vi "Display Module Refresh Rate.vi"(7 "Refresh Rate In":u32) -> (8 "Refresh Rate Out":u32)   [LabVIEW 2020]
uses:
  <vilib>/Utility/miscctls.llb/LVPointTypeDef.ctl
panel:
  in  "Refresh Rate (ms)":u32
  in  "Cancel":bool
  in  "Okay":bool
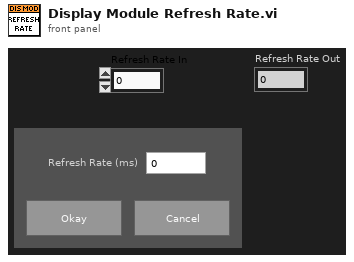
[diagram p1: front panel]
types:
  T1 = enum16{"Always On", "Always Off", "Off While Running"}
  T2 = typedef "LVPointTypeDef.ctl" = cluster{"Horizontal":i16, "Vertical":i16}
  T3 = typedef "LVRectTypeDef.ctl" = cluster{"Left":i16, "Top":i16, "Right":i16, "Bottom":i16}
  T4 = typedef "LVBoundsTypeDef.ctl" = cluster{"Width":u32, "Height":u32}
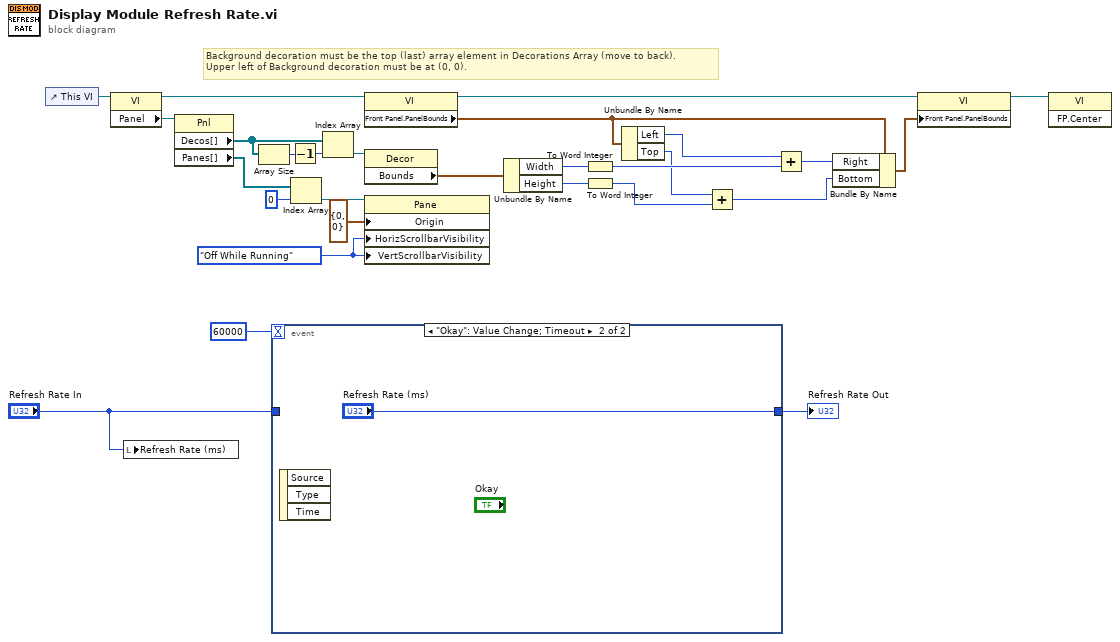
[diagram p0: block diagram]
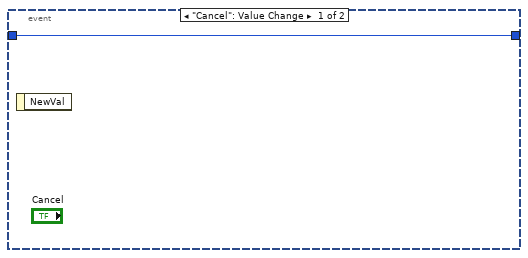
[diagram p2: hidden frame]
diagram:
  w16 = T1."Off While Running" ("Vertical Scrollbar Visibility")
  # "Background decoration must be the top (last) array element in Decorations Array (move to back).\nUpper left of Background decoration must be at (0, 0)."
  n1 = control-ref of="This VI"() -> (w9:refnum<vi>)
  n2 = property class="VI"(reference=w9) -> (reference out=w17:refnum<vi>, "Panel"=w10:refnum<vi>)  [unwired: 1 in, 1 out]
  n3 = local write "Refresh Rate (ms)"("Refresh Rate In") -> ()
  n4 = property class="Pnl"(reference=w10) -> ("Decos[]"=w8:refnum<vi>[], "Panes[]"=w13:refnum<vi>[])  [unwired: 1 in, 2 out]
  n5 = Array Size(array=w8) -> (size(s)=w6:i32)
  n6 = event shown="[1] \"Okay\": Value Change;  Timeout" {
    selector: _ -> [_ _]
    dyn-events: _ -> [_ _]
    timeout: 60000 -> [_ _]
    tunnel: "Refresh Rate In" -> [w29 _]
    tunnel: [w29 "Refresh Rate (ms)"] -> w27
    event "Cancel": Value Change {
      n7 = event-data() -> ()  [unwired: 1 in, 1 out]
    }
    event "Okay": Value Change; Timeout {
      n8 = event-data() -> ()  [unwired: 1 in, 3 out]
    }
  }
  "Refresh Rate Out" <- w27
  n9 = Decrement(x=w6) -> (x-1=w7:i32)
  n10 = Index Array(array=w13, index=0) -> (element=w12:refnum<vi>)
  n11 = Index Array(array=w8, index=w7) -> (element=w15:refnum<vi>)
  n12 = property class="VI"(reference=w17) -> (reference out=w19:refnum<vi>, "Front Panel.PanelBounds"=w20:T3)  [unwired: 1 in, 1 out]
  n13 = property class="Decor"(reference=w15) -> ("Bounds"=w18:T4)  [unwired: 1 in, 2 out]
  n14 = property class="Pane"(reference=w12, "Origin"=T2 {"Horizontal"=0, "Vertical"=0}, "HorizScrollbarVisibility"=w16, "VertScrollbarVisibility"=w16) -> ()  [unwired: 1 in, 2 out]
  n15 = Unbundle By Name(w18) -> ("Width"=w23:u32, "Height"=w26:u32)
  n16 = To Word Integer(number=w23) -> (16bit integer=w25:i16)
  n17 = To Word Integer(number=w26) -> (16bit integer=w4:i16)
  n18 = Unbundle By Name(w20) -> ("Left"=w22:i16, "Top"=w5:i16)
  n19 = Add(x=w5, y=w4) -> (x+y=w3:i16)
  n20 = Add(x=w22, y=w25) -> (x+y=w24:i16)
  n21 = Bundle By Name(cluster=w20, "Right"=w24, "Bottom"=w3) -> (w21:T3)
  n22 = property class="VI"(reference=w19, "Front Panel.PanelBounds"=w21) -> (reference out=w2:refnum<vi>)  [unwired: 1 in, 1 out]
  n23 = invoke class="VI" method="FP.Center"(reference=w2) -> ()  [unwired: 2 in, 3 out]
